vi "Generic command handler.vi"(8 "error in (no error)":errorcluster, 10 "Message in":refnum<class "GenericMessage.lvclass">, 11 "Galvo in":refnum<class "ImagingModeSPIM.lvclass">) -> (0 "error out":errorcluster, 2 "value":string, 3 "Galvo out":refnum<class "ImagingModeSPIM.lvclass">)   [LabVIEW 2012, in "ImagingModeSPIM.lvclass"]
doc: "The generic_command_handler processes the command 'generic'. Commands which are not part of the predefined list of commands fall under the 'generic' command for special activity."
uses:
  ImagingModeSPIM.lvclass
  ImagingModeFlexTrajectoryScaffold/ImagingModeFlexTrajectoryScaffold/ImagingModeFlexTrajectoryScaffold.lvclass
  <vilib>/Distrio/Murmex/GenericMessage/GenericMessage.lvclass
panel:
  # "This method is called when the GENERIC\ntrigger is sent. \n\nOverride this method when your component needs to\nrespond to this trigger. \n\nCall parent for proper implementation"
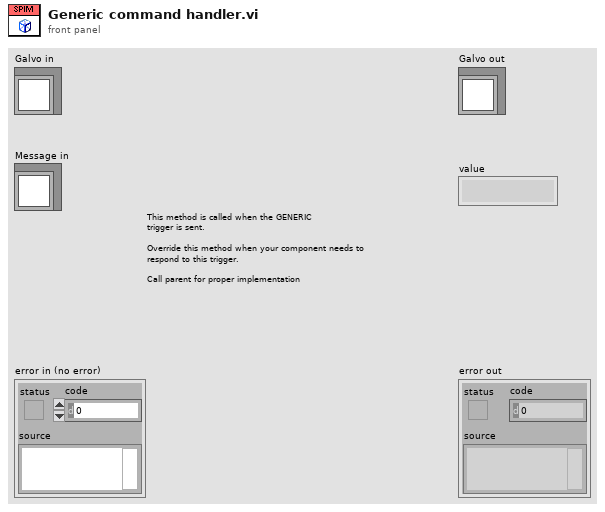
[diagram p1: front panel]
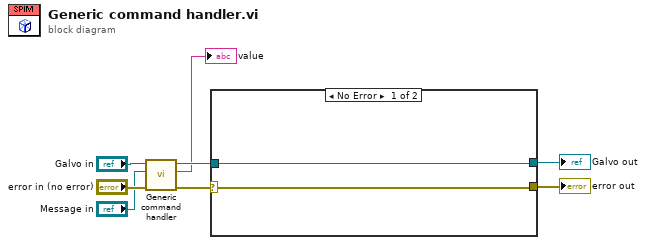
[diagram p0: block diagram]
diagram:
  n1 = call-parent "Generic command handler.vi"("error in (no error)"="error in (no error)", "Message in"="Message in", "ImagingModeDL090130Frame in"="Galvo in") -> ("error out"=w6:errorcluster, "value"=→"value":string, "ImagingModeDL090130Frame out"=w5:refnum<class "ImagingModeSPIM.lvclass">)  [unwired: 6 in]
  n2 = case shown="No Error" w6 {
    selector: w6 -> [w9 w11]
    tunnel: w5 -> [w10 w12]
    tunnel: [w9 w11] -> w3
    tunnel: [w10 w12] -> w2
    frame No Error {
    }
    frame Error {
    }
  }
  "error out" <- w3
  "Galvo out" <- w2
